vi "checkFinishPassPlay.vi"(8 "error in (no error)":errorcluster, 10 "Game":refnum<class "Game.lvclass">, 11 "PassPlay in":refnum<class "PassPlay.lvclass">) -> (0 "error out":errorcluster, 2 "Boolean":bool, 3 "PassPlay out":refnum<class "PassPlay.lvclass">)   [LabVIEW 2024, in "PassPlay.lvclass"]
uses:
  PassPlay.lvclass
  Game_class/Game.lvclass
  Referee_class/command_interpreted.ctl
  Ball_class/Ball.lvclass
  Game_class/Game.lvclass/Game.ctl
  Referee_class/Referee.lvclass/Referee.ctl
  Events_class/Events.lvclass/Events.ctl
  Team_class/Team.lvclass/Team.ctl
  Game_class/Read Referee.vi
  Game_class/Read EventsRef.vi
  Game_class/Read Utilities.lvclass.vi
  Game_class/Read AllyRef.vi
  Game_class/Read EnemyRef.vi
  Team_class/Read RobotRef.vi
  Events_class/Read ball_out.vi
  Events_class/Read touch.vi
  Referee_class/Read command_interpreted.vi
  Enemy_class/Enemy.lvclass
  C:/Users/moise/Documents/GitHub/SSL_AI/Team_class/Team.lvclass
  Ally_class/Ally.lvclass
  Referee_class/Referee.lvclass
  Events_class/Events.lvclass
  Utilities_class/Utilities.lvclass
  Robot_class/Robot.lvclass
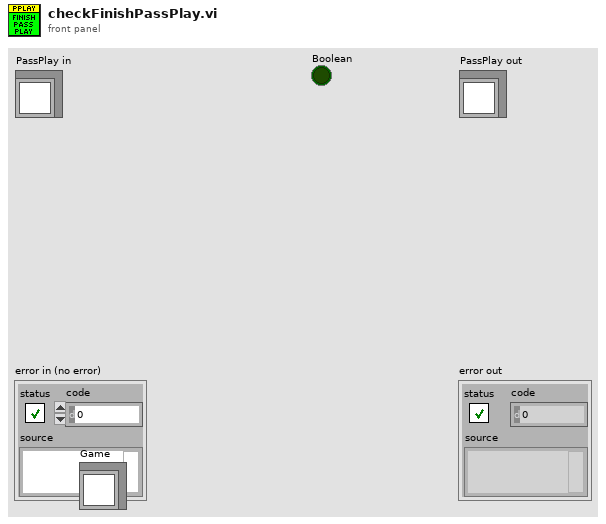
[diagram p1: front panel]
types:
  T1 = typedef "command_interpreted.ctl" = enum16{"Goal Ally", "Goal Enemy", "Ball Placement Enemy", "Ball Placement Ally", "Normal Half Time", "Extra Time  Break", "Extra Half Time", "None", "Post Game", "PKA Normal Start", "Prepare Kickoff Ally", "PKE Normal Start", "Prepare Kickoff Enemy", "Force Start", "Halt", "Timeout", "Prepare Penalty Ally", "Prepare Penalty Enemy", "PPA NormalStart", "PPE Normal Start", "Indirect Free Ally", "Direct Free Enemy", "Direct Free Ally", "Indirect Free Enemy", "Stop"}
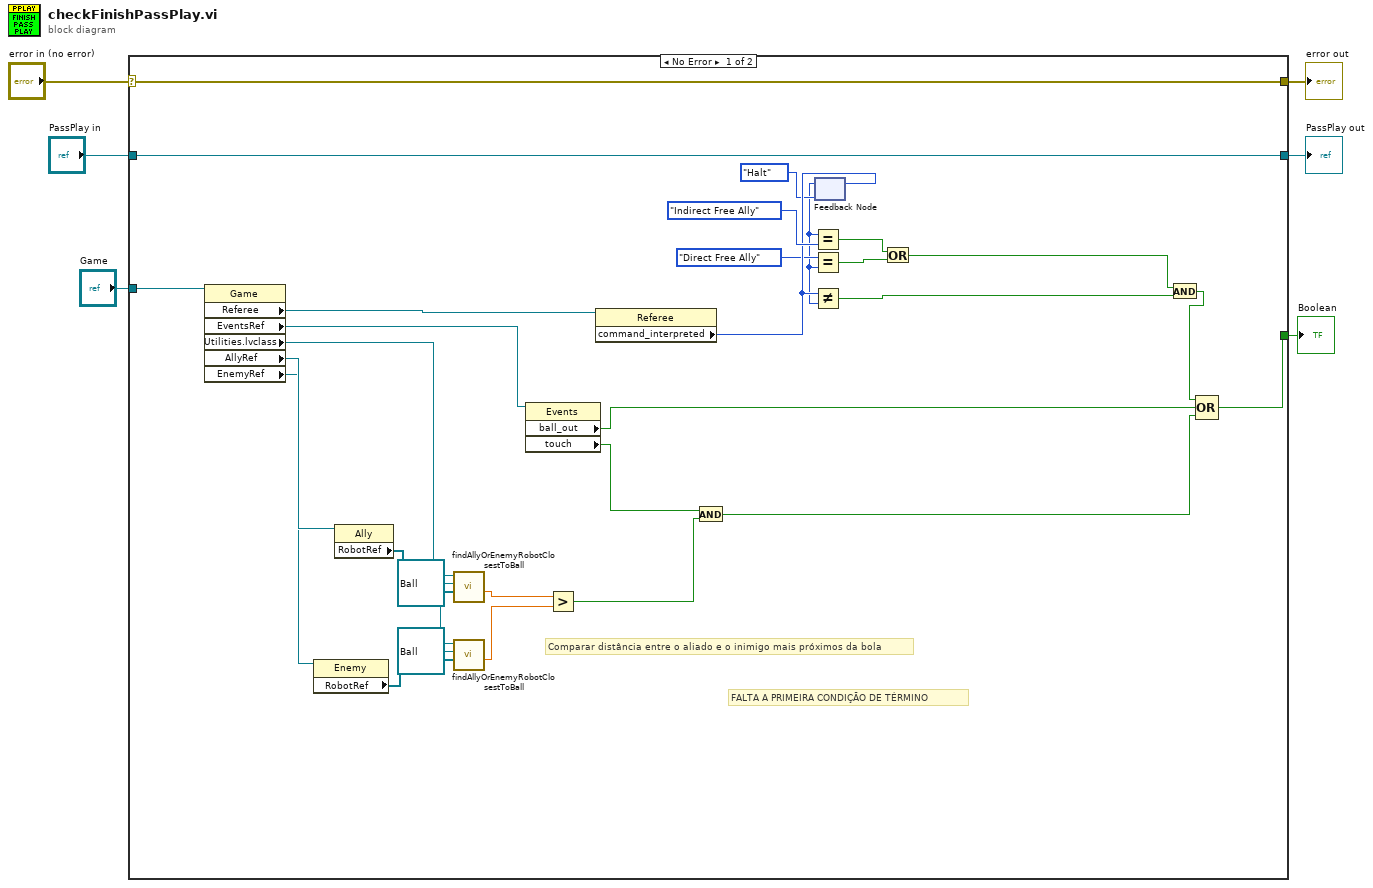
[diagram p0: block diagram]
diagram:
  n1 = case shown="No Error" "error in (no error)" {
    selector: "error in (no error)" -> [w34 w37]
    tunnel: [w34 w37] -> w5
    tunnel: [w35 w36] -> w3
    tunnel: "PassPlay in" -> [w35 w36]
    tunnel: "Game" -> [w18 _]
    tunnel: [w20 _] -> w1
    frame No Error {
      # "Comparar distância entre o aliado e o inimigo mais próximos da bola"
      # "FALTA A PRIMEIRA CONDIÇÃO DE TÉRMINO"
      n2 = property class="Game"(reference=w18) -> ("Referee"=w33:refnum<class "Referee.lvclass">, "EventsRef"=w23:refnum<class "Events.lvclass">, "Utilities.lvclass"=w19:refnum<class "Utilities.lvclass">, "AllyRef"=w17:refnum<class "Ally.lvclass">, "EnemyRef"=w16:refnum<class "Enemy.lvclass">)  [unwired: 1 in, 2 out]
      n3 = property class="Enemy"(reference=w16) -> ("RobotRef"=w14:refnum<class "Robot.lvclass">[])  [unwired: 1 in, 2 out]
      n4 = property class="Ally"(reference=w17) -> ("RobotRef"=w15:refnum<class "Robot.lvclass">[])  [unwired: 1 in, 2 out]
      n5 = call "findAllyOrEnemyRobotClosestToBall.vi"("Ally/Enemy Robots"=w15, "Ball"=refnum<class "Ball.lvclass"> refnum, "Utilities in"=w19) -> ("Robot distance to ball"=w12:dbl)  [unwired: 4 in, 4 out]
      n6 = call "findAllyOrEnemyRobotClosestToBall.vi"("Ally/Enemy Robots"=w14, "Ball"=refnum<class "Ball.lvclass"> refnum, "Utilities in"=w19) -> ("Robot distance to ball"=w11:dbl)  [unwired: 4 in, 4 out]
      n7 = property class="Events"(reference=w23) -> ("ball_out"=w21:bool, "touch"=w13:bool)  [unwired: 1 in, 2 out]
      n8 = Greater?(x=w12, y=w11) -> (0:w10:bool)
      n9 = property class="Referee"(reference=w33) -> ("command_interpreted"=w31:T1)  [unwired: 1 in, 2 out]
      n10 = And(x=w13, y=w10) -> (x .and. y?=w9:bool)
      n11 = feedback #1(command_interpreted."Halt" ("command_interpreted")) -> (w27:T1)
      n12 = Equal?(x=w27, y=command_interpreted."Indirect Free Ally" ("command_interpreted")) -> (x = y?=w25:bool)
      n13 = Equal?(x=command_interpreted."Direct Free Ally" ("command_interpreted"), y=w27) -> (x = y?=w26:bool)
      n14 = Not Equal?(x=w31, y=w27) -> (x != y?=w30:bool)
      n15 = feedback-in #1(w31) -> ()
      n16 = Or(x=w25, y=w26) -> (x .or. y?=w24:bool)
      n17 = And(x=w24, y=w30) -> (x .and. y?=w22:bool)
      n18 = Compound Arithmetic op=OR(w22, w21, w9) -> (w20:bool)
    }
    frame Error {
    }
  }
  "error out" <- w5
  "PassPlay out" <- w3
  "Boolean" <- w1
